vi "raised_cos_sigmoid.vi"(8 "B":dbl, 9 "A":dbl, 11 "x":dbl) -> (3 "raised_cos_sigmoid(x, A, B)":dbl)   [LabVIEW 2019]
panel:
  # "REQUIRE: A <= B. This VI is not robust, it will not raise an exception if this requirement is violated."
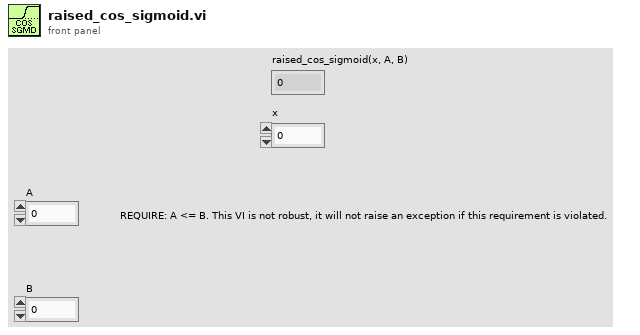
[diagram p1: front panel]
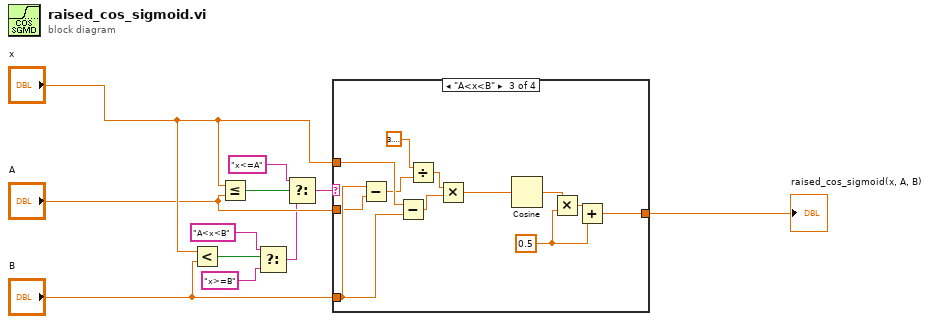
[diagram p0: block diagram]
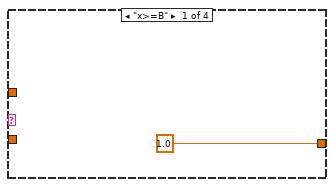
[diagram p2: hidden frame]
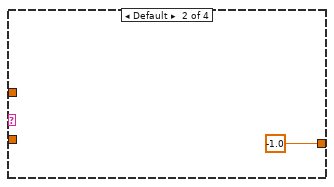
[diagram p3: hidden frame]
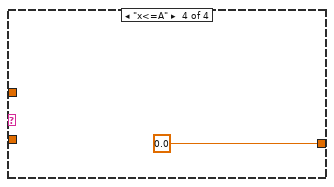
[diagram p4: hidden frame]
diagram:
  n1 = Less?(x="x", y="B") -> (x < y?=w3:bool)
  n2 = Less Or Equal?(x="x", y="A") -> (x <= y?=w5:bool)
  n3 = Select(t="A<x<B", s=w3, f="x>=B") -> (s? t:f=w7:string)
  n4 = Select(t="x<=A", s=w5, f=w7) -> (s? t:f=w6:string)
  n5 = case shown="\"A<x<B\"" w6 {
    tunnel: [1.0 -1.0 w14 0.0] -> w8
    tunnel: "x" -> [_ _ w22 _]
    tunnel: "B" -> [_ _ w19 _]
    tunnel: "A" -> [_ _ w18 _]
    frame "x>=B" {
    }
    frame Default {
    }
    frame "A<x<B" {
      w24 = 0.5
      n6 = Subtract(x=w19, y=w18) -> (x-y=w20:dbl)
      n7 = Subtract(x=w22, y=w19) -> (x-y=w21:dbl)
      n8 = Divide(x=3.141592653589793, y=w20) -> (x/y=w16:dbl)
      n9 = Multiply(x=w16, y=w21) -> (x*y=w15:dbl)
      n10 = Cosine(x=w15) -> (cos(x)=w23:dbl)
      n11 = Multiply(x=w23, y=w24) -> (x*y=w25:dbl)
      n12 = Add(x=w25, y=w24) -> (x+y=w14:dbl)
    }
    frame "x<=A" {
    }
  }
  "raised_cos_sigmoid(x, A, B)" <- w8
